vi "Check FP Window Size.vi"(4 "Default Height":i16, 6 "Default Width":i16, 9 "Display:All Monitors":T1, 10 "FP.WinBounds":T2, 11 "Default":T2) -> (2 "Use Default Values":bool, 3 "FP.WinBounds out":T2)   [LabVIEW 2017, in "Settings.lvclass"]
uses:
  Settings.lvclass
  <vilib>/Utility/miscctls.llb/LVRectTypeDef.ctl
  <vilib>/Utility/miscctls.llb/LVAllMonitorsDisplayTypeDef.ctl
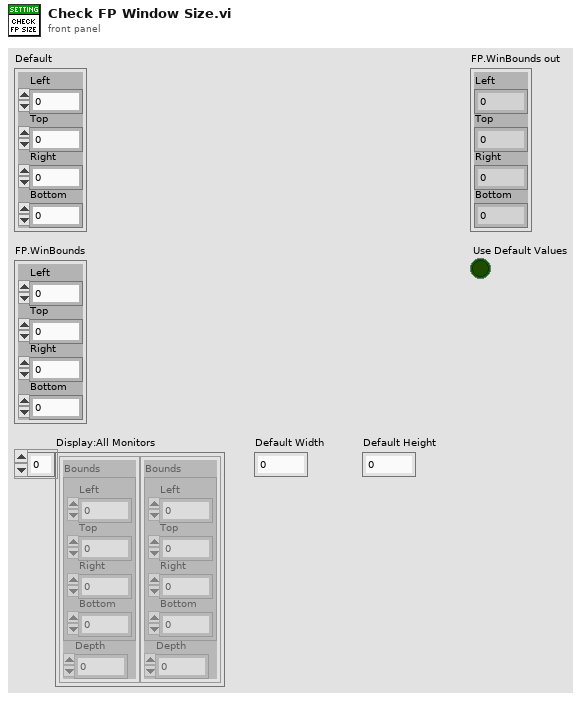
[diagram p1: front panel]
types:
  T1 = typedef "LVAllMonitorsDisplayTypeDef.ctl" = cluster{"Bounds":cluster{"Left":i16, "Top":i16, "Right":i16, "Bottom":i16}, "Depth":i16}[]
  T2 = typedef "LVRectTypeDef.ctl" = cluster{"Left":i16, "Top":i16, "Right":i16, "Bottom":i16}
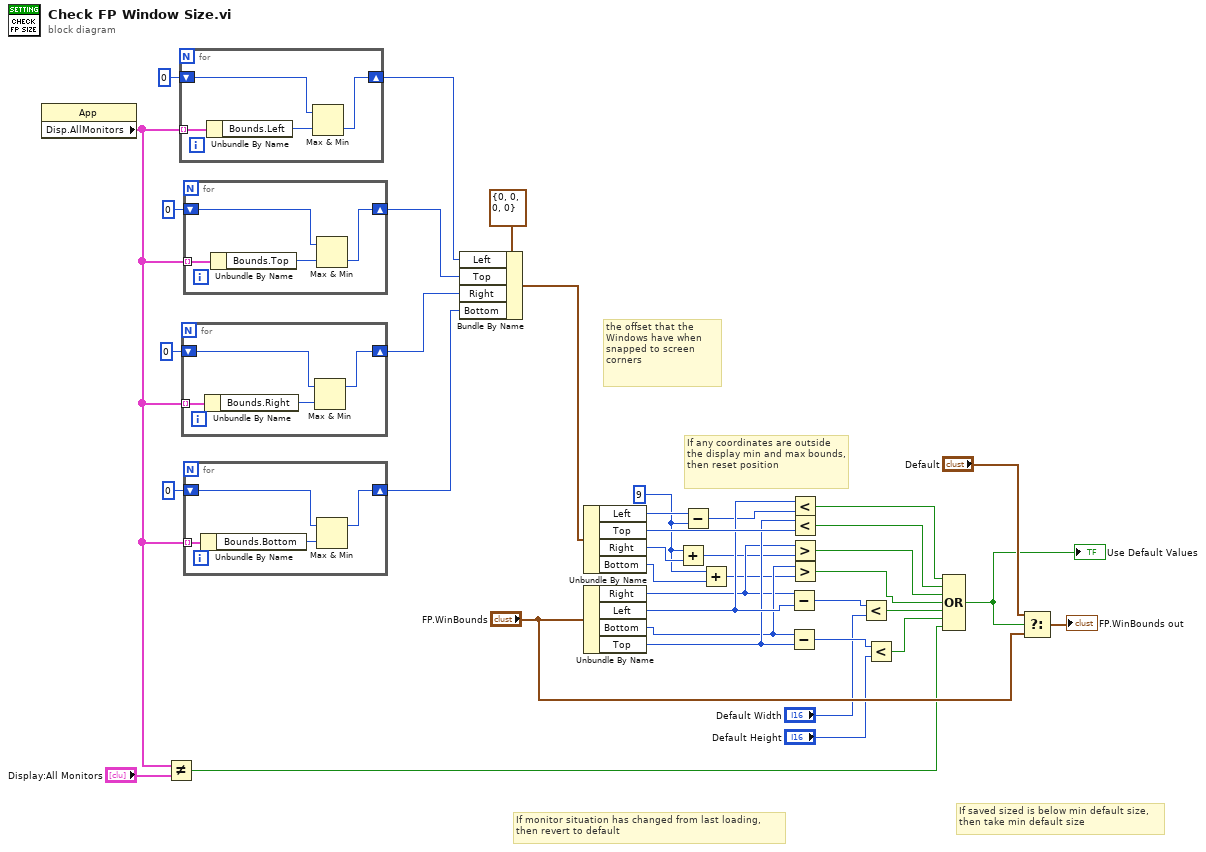
[diagram p0: block diagram]
diagram:
  w3 = i16 9 ("x")
  # "If saved sized is below min default size,\nthen take min default size"
  # "the offset that the Windows have when snapped to screen corners"
  # "If monitor situation has changed from last loading,\nthen revert to default"
  # "If any coordinates are outside the display min and max bounds, then reset position"
  n1 = property class="App"() -> ("Disp.AllMonitors"=w9:T1)  [unwired: 2 in, 2 out]
  n2 = Not Equal?(x=w9, y="Display:All Monitors") -> (x != y?=w8:bool)
  n3 = for {
    tunnel: w9 -> [w43] mode=indexing
    shift-right: [w40] -> w14
    shift-left: i16 0 ("Bounds.Left") -> [w42]
    n4 = Unbundle By Name(w43) -> ("Bounds.Left"=w41:i16)
    n5 = Max & Min(x=w42, y=w41) -> (min(x,y)=w40:i16)  [unwired: 1 out]
  }
  n6 = for {
    tunnel: w9 -> [w47] mode=indexing
    shift-right: [w44] -> w12
    shift-left: i16 0 ("Bounds.Left") -> [w46]
    n7 = Unbundle By Name(w47) -> ("Bounds.Right"=w45:i16)
    n8 = Max & Min(x=w46, y=w45) -> (max(x,y)=w44:i16)  [unwired: 1 out]
  }
  n9 = for {
    tunnel: w9 -> [w51] mode=indexing
    shift-right: [w48] -> w13
    shift-left: i16 0 ("Bounds.Left") -> [w50]
    n10 = Unbundle By Name(w51) -> ("Bounds.Top"=w49:i16)
    n11 = Max & Min(x=w50, y=w49) -> (min(x,y)=w48:i16)  [unwired: 1 out]
  }
  n12 = for {
    tunnel: w9 -> [w55] mode=indexing
    shift-right: [w52] -> w11
    shift-left: i16 0 ("Bounds.Left") -> [w54]
    n13 = Unbundle By Name(w55) -> ("Bounds.Bottom"=w53:i16)
    n14 = Max & Min(x=w54, y=w53) -> (max(x,y)=w52:i16)  [unwired: 1 out]
  }
  n15 = Bundle By Name(cluster=T2 {"Left"=0, "Top"=0, "Right"=0, "Bottom"=0} ("input cluster"), "Left"=w14, "Top"=w13, "Right"=w12, "Bottom"=w11) -> (w15:T2)
  n16 = Unbundle By Name(w15) -> ("Left"=w32:i16, "Top"=w31:i16, "Right"=w29:i16, "Bottom"=w27:i16)
  n17 = Unbundle By Name("FP.WinBounds") -> ("Right"=w6:i16, "Left"=w30:i16, "Bottom"=w7:i16, "Top"=w28:i16)
  n18 = Add(x=w3, y=w29) -> (x+y=w5:i16)
  n19 = Subtract(x=w32, y=w3) -> (x-y=w21:i16)
  n20 = Add(x=w3, y=w27) -> (x+y=w4:i16)
  n21 = Subtract(x=w6, y=w30) -> (x-y=w39:i16)
  n22 = Subtract(x=w7, y=w28) -> (x-y=w38:i16)
  n23 = Less?(x=w30, y=w21) -> (x < y?=w26:bool)
  n24 = Less?(x=w28, y=w31) -> (x < y?=w25:bool)
  n25 = Greater?(x=w6, y=w5) -> (0:w24:bool)
  n26 = Greater?(x=w7, y=w4) -> (0:w23:bool)
  n27 = Less?(x=w39, y="Default Width") -> (x < y?=w33:bool)
  n28 = Less?(x=w38, y="Default Height") -> (x < y?=w34:bool)
  n29 = Compound Arithmetic op=OR(w26, w25, w24, w23, w33, w34, w8) -> (w22:bool)
  "Use Default Values" <- w22
  n30 = Select(t="Default", s=w22, f="FP.WinBounds") -> (s? t:f=→"FP.WinBounds out":T2)
